vi "CloseProgressBar.vi"(8 "error in (no error)":errorcluster, 11 "VI Refnum":refnum<vi>) -> (0 "error out":errorcluster)   [LabVIEW 2017]
panel:
  out "error out 2":errorcluster
  in  "error in (no error) 2":errorcluster
  in  "reference in":refnum<vi>
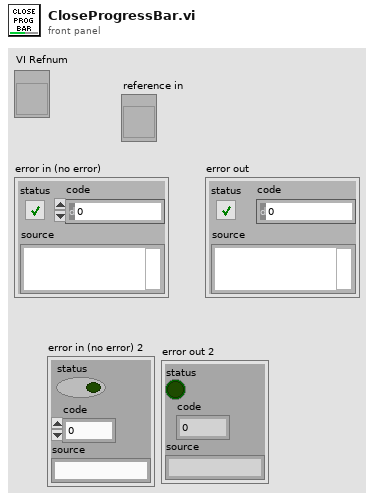
[diagram p1: front panel]
types:
  T1 = enum32{"Invalid", "Standard", "Closed", "Hidden", "Minimized", "Maximized"}
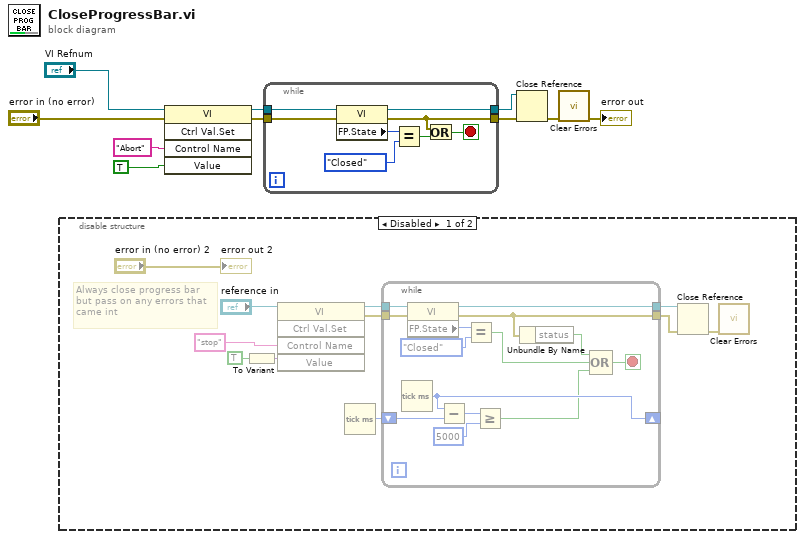
[diagram p0: block diagram]
diagram:
  n1 = disable-structure shown="Disabled" {
    frame Disabled {
      # "Always close progress bar\nbut pass on any errors that\ncame int"
      n2 = To Variant(anything=TRUE) -> (Variant=w18:variant)
      n3 = invoke class="VI" method="Ctrl Val.Set"(reference="reference in", "Control Name"="stop", "Value"=w18) -> (reference out=w16:refnum<vi>, error out=w14:errorcluster)  [unwired: 2 in, 3 out]
      n4 = Tick Count (ms)() -> (millisecond timer value=w11:u32)
      n5 = while {
        tunnel: w16 -> [w35]
        tunnel: [w34] -> w15
        tunnel: w14 -> [w31]
        tunnel: [w30] -> w13
        shift-right: [w25] -> _
        shift-left: w11 -> [w26]
        stop <- w28 stop-if-true
        n6 = Tick Count (ms)() -> (millisecond timer value=w25:u32)
        n7 = property class="VI"(reference=w35, error in=w31) -> (reference out=w34:refnum<vi>, error out=w30:errorcluster, "FP.State"=w33:T1)
        n8 = Subtract(x=w25, y=w26) -> (x-y=w24:u32)
        n9 = Equal?(x=w33, y=T1."Closed") -> (x = y?=w29:bool)
        n10 = Greater Or Equal?(x=w24, y=u32 5000) -> (x >= y?=w22:bool)
        n11 = Unbundle By Name(w30) -> ("status"=w27:bool)
        n12 = Compound Arithmetic op=OR(w27, w29, w22) -> (w28:bool)
      }
      n13 = Close Reference(reference=w15, error in (no error)=w13) -> (error out=w12:errorcluster)
      n14 = call <vilib>:"Clear Errors.vi"("error in (no error)"=w12) -> ()  [unwired: 5 in, 2 out]
      "error out 2" <- "error in (no error) 2"
    }
    frame Enabled {
    }
  }
  n15 = invoke class="VI" method="Ctrl Val.Set"(reference="VI Refnum", error in="error in (no error)", "Control Name"="Abort", "Value"=TRUE) -> (reference out=w7:refnum<vi>, error out=w6:errorcluster)  [unwired: 1 in, 3 out]
  n16 = while {
    tunnel: w7 -> [w43]
    tunnel: w6 -> [w42]
    tunnel: [w37] -> w5
    tunnel: [w36] -> w4
    stop <- w38 stop-if-true
    n17 = property class="VI"(reference=w43, error in=w42) -> (reference out=w37:refnum<vi>, error out=w36:errorcluster, "FP.State"=w41:T1)
    n18 = Equal?(x=w41, y=T1."Closed" ("Front Panel Window:State")) -> (x = y?=w39:bool)
    n19 = Or(x=w36, y=w39) -> (x .or. y?=w38:bool)
  }
  n20 = Close Reference(reference=w5, error in (no error)=w4) -> (error out=w2:errorcluster)
  n21 = call <vilib>:"Clear Errors.vi"("error in (no error)"=w2) -> ("error out"=→"error out":errorcluster)  [unwired: 5 in, 1 out]
